vi "Vision Processing.vi"() -> ()   [LabVIEW 2011]
doc: "This VI runs in parallel to other tasks. It gets images from the camera, processes them for color or shape and use that information to affect robot behavior."
uses:
  Robot Global Data.vi
  <vilib>/vision/NI_Vision_Development_Module.lvlib
panel:
  out "Midpoint":dbl
  in  "Lower Speed Limit":dbl=0.05
  out "Turret Rotation":dbl
  in  "Upper Speed Limit":dbl=0.3
  out "Number of Rectangles Visible":dbl
  out "Y Position Array":dbl[](array[numeric])
  out "X Position Array":dbl[](array[numeric])
  out "Array":T1(array[cluster])
  in  "Score Limits":T2={"Rect Coverage"=76.0, "Aspect Ratio"=40.0, "X Edge Strength"=40.0, "Y Edge Strength"=60.0}
  out "Processed Image":T3(plugin-control)
  out "Original Image":T3(plugin-control)
  in  "Annotate":bool=TRUE
  in  "Particle Count Limit":i32=10
  in  "Area Size Limit":i32=444
  in  "Range":cluster{"Lower value":sgl, "Upper value":sgl}={"Lower value"=120.0, "Upper value"=255.0}
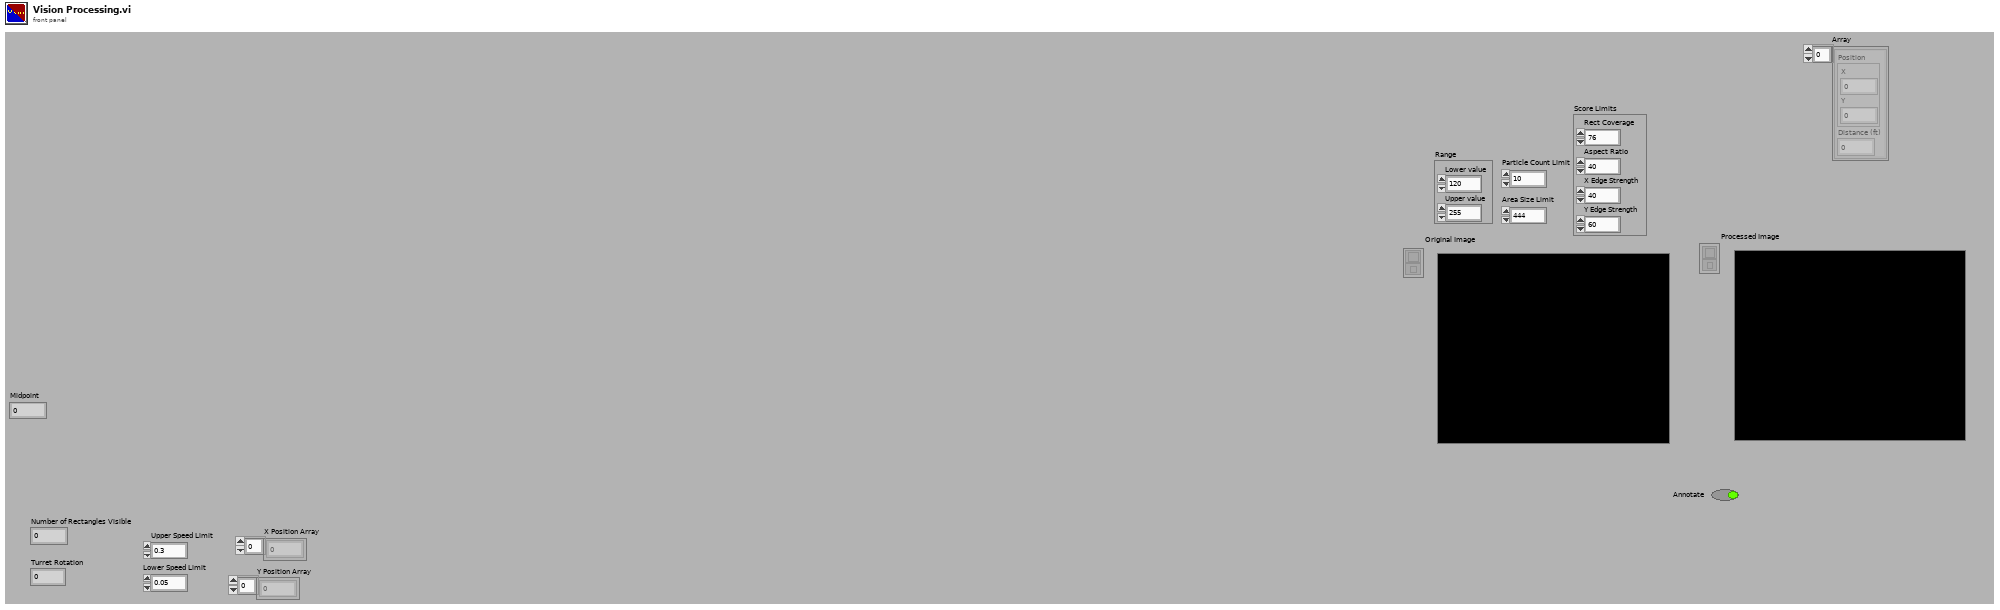
[diagram p1: front panel]
types:
  T1 = cluster{"Position":cluster{"X":dbl, "Y":dbl}, "Distance (ft)":dbl}[]
  T2 = cluster{"Rect Coverage":dbl, "Aspect Ratio":dbl, "X Edge Strength":dbl, "Y Edge Strength":dbl}
  T3 = typedef "IMAQ Image.ctl" = refnum<image>
  T4 = typedef "Image Type" = u32
  T5 = typedef "WPI_CameraImageSize.ctl" = enum16{"640x480", "320x240", "160x120"}
  T6 = cluster{"fps":i32, "compression":i32, "Image Size":T5}
  T7 = cluster{cluster{"Left":dbl, "Top":dbl, "Right":dbl, "Bottom":dbl}, dbl[]}[]
  T8 = cluster{"Left":dbl, "Top":dbl, "Right":dbl, "Bottom":dbl}
  T9 = cluster{"Target Center (-1 to 1)":cluster{"X":dbl, "Y":dbl}, "Distance (ft)":dbl}
  T10 = cluster{"Target Center (-1 to 1)":cluster{"X":dbl, "Y":dbl}, "Distance (ft)":dbl}[]
  T11 = cluster{"Axis 1":dbl, "Axis 2":dbl, "Axis 3":dbl, "Axis 4":dbl, "Axis 5":dbl, "Axis 6":dbl, "Button 1":bool, "Button 2":bool, "Button 3":bool, "Button 4":bool, "Button 5":bool, "Button 6":bool, "Button 7":bool, "Button 8":bool, "Button 9":bool, "Button 10":bool, "Button 11":bool, "Button 12":bool}
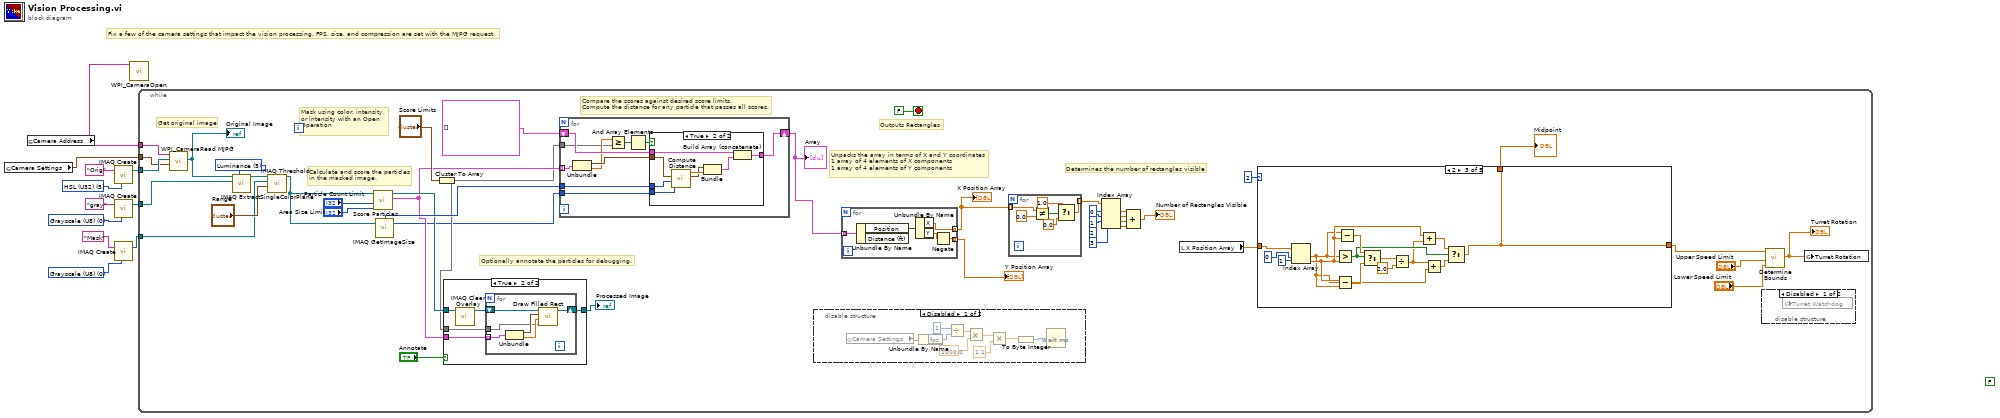
[diagram p0: block diagram]
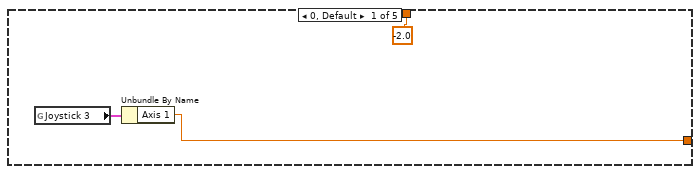
[diagram p4: hidden frame]
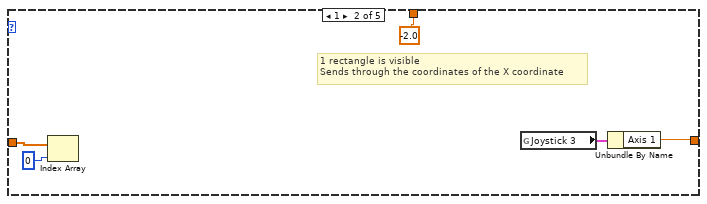
[diagram p5: hidden frame]
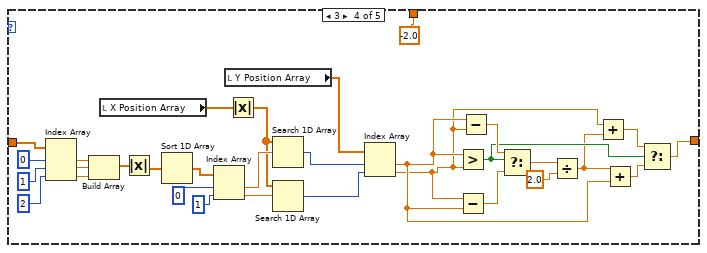
[diagram p6: hidden frame]
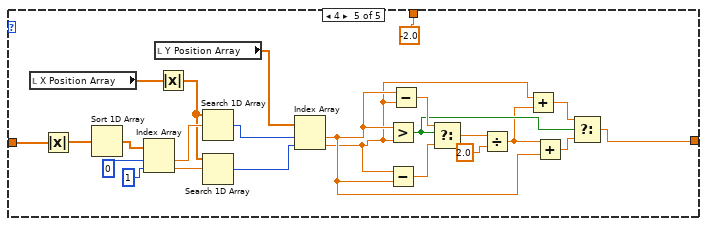
[diagram p7: hidden frame]
diagram:
  (unwired) FALSE
  w4 = T4 0 items=["Grayscale (U8)", "Grayscale (I16)", "Grayscale (SGL)", "Complex (CSG)", "RGB (U32)", "HSL (U32)", "RGB (U64)", "Grayscale (U16)"] ("Image Type")
  w8 = T4 5 items=["Grayscale (U8)", "Grayscale (I16)", "Grayscale (SGL)", "Complex (CSG)", "RGB (U32)", "HSL (U32)", "RGB (U64)", "Grayscale (U16)"] ("Image Type")
  w11 = T4 0 items=["Grayscale (U8)", "Grayscale (I16)", "Grayscale (SGL)", "Complex (CSG)", "RGB (U32)", "HSL (U32)", "RGB (U64)", "Grayscale (U16)"] ("Image Type")
  # "Fix a few of the camera settings that impact the vision processing. FPS, size, and compression are set with the MJPG request."
  n1 = global read "Robot Global Data.vi" "Camera Settings"() -> (w1:T6)
  n2 = global read "Robot Global Data.vi" "Camera Address"() -> (w2:string)
  n3 = call "IMAQ Create"("Image Name"="Orig", "Image Type"=w8) -> ("New Image"=w7:T3)  [unwired: 2 in, 2 out]
  n4 = call "IMAQ Create"("Image Name"="gray", "Image Type"=w11) -> ("New Image"=w6:T3)  [unwired: 2 in, 2 out]
  n5 = call "IMAQ Create"("Image Name"="Mask", "Image Type"=w4) -> ("New Image"=w3:T3)  [unwired: 2 in, 2 out]
  n6 = call <vilib>:"WPI_CameraOpen.vi"("Camera Address"=w2) -> ()  [unwired: 9 in, 2 out]
  n7 = while {
    tunnel: w7 -> [w52]
    tunnel: w6 -> [w34]
    tunnel: w3 -> [w36]
    tunnel: w2 -> [w51]
    tunnel: w1 -> [w40]
    stop <- FALSE stop-if-true
    w39 = 5 items=["Red", "Green", "Blue", "Hue", "Saturation", "Luminance", "Value", "Intensity"] ("Color Plane")
    # "Determines the number of rectangles visible"
    # "Unpacks the array in terms of X and Y coordinates\n1 array of 4 elements of X components\n1 array of 4 elements of Y components"
    # "Outputs Rectangles"
    # "Optionally annotate the particles for debugging."
    # "Compare the scores against desired score limits.\nCompute the distance for any particle that passes all scores."
    # "Calculate and score the particles\nin the masked image."
    # "Mask using color, intensity,\nor intensity with an Open\nOperation"
    # "Get original image"
    n8 = call <vilib>:"WPI_CameraRead MJPG.vi"("Camera Settings"=w40, "Image"=w52, "address"=w51) -> ("Image Out"=w35:T3)  [unwired: 7 in, 1 out]
    "Original Image" <- w35
    n9 = call "IMAQ ExtractSingleColorPlane"("Color Plane"=w39, "Image Dst"=w34, "Image Src"=w35) -> ("Image Dst Out"=w37:T3)  [unwired: 1 in, 7 out]
    n10 = call "IMAQ Threshold"("Range"="Range", "Image Dst"=w36, "Image Src"=w37) -> ("Image Dst Out"=w33:T3)  [unwired: 3 in, 5 out]
    n11 = call "Score Particles.vi"("Area Size Limit"="Area Size Limit", "Particle Count Limit"="Particle Count Limit", "Image Refnum in"=w33) -> ("Scored Particle Info"=w47:T7, "Image Refnum out"=w50:T3)  [unwired: 7 in]
    n12 = call "IMAQ GetImageSize"("Image"=w33) -> ("Y Resolution"=w41:i32, "X Resolution"=w53:i32)  [unwired: 3 in, 1 out]
    n13 = Cluster To Array(cluster="Score Limits") -> (array=w45:dbl[])
    n14 = case shown="True" "Annotate" {
      tunnel: w50 -> [w151 w156]
      tunnel: [w151 w155] -> w48
      tunnel: w47 -> [_ w153]
      tunnel: w45 -> [_ w152]
      frame False {
      }
      frame True {
        n15 = call "IMAQ Clear Overlay"("Image"=w156) -> ("Image Out"=w154:T3)  [unwired: 2 in, 8 out]
        n16 = for {
          shift-right: [w161] -> w155
          shift-left: w154 -> [w162]
          tunnel: w153 -> [w158] mode=indexing
          tunnel: w152 -> [w157]
          n17 = Unbundle(w158) -> (w159:T8, w160:dbl[])
          n18 = call "Draw Filled Rect.vi"("Limits"=w157, "Scores"=w160, "Bounding Box"=w159, "image in"=w162) -> ("image out"=w161:T3)  [unwired: 7 in]
        }
      }
    }
    "Processed Image" <- w48
    n19 = for {
      shift-right: [w171] -> w12
      shift-left: T1 [] -> [w172]
      tunnel: w53 -> [w170]
      tunnel: w47 -> [w168] mode=indexing
      tunnel: w45 -> [w164]
      tunnel: w41 -> [w163]
      n20 = Unbundle(w168) -> (w169:T8, w165:dbl[])
      n21 = Greater Or Equal?(x=w165, y=w164) -> (x >= y?=w167:bool[])
      n22 = And Array Elements(Boolean array=w167) -> (logical AND=w166:bool)
      n23 = case shown="True" w166 {
        tunnel: w172 -> [w173 w181]
        tunnel: [w173 w180] -> w171
        tunnel: w169 -> [_ w176]
        tunnel: w170 -> [_ w178]
        tunnel: w163 -> [_ w174]
        frame False {
        }
        frame True {
          n24 = call "Compute Distance.vi"("Y Image Resolution"=w174, "X Image Resolution"=w178, "Bounding Box"=w176) -> ("Target Center (-1 to 1)"=w175:cluster{"X":dbl, "Y":dbl}, "Distance (ft)"=w177:dbl)  [unwired: 7 in]
          n25 = Bundle("Target Center (-1 to 1)"=w175, "Distance (ft)"=w177) -> (w179:T9)  [unwired: 1 in]
          n26 = Build Array (concatenate)(w181, w179) -> (w180:T10)
        }
      }
    }
    "Array" <- w12
    n27 = disable-structure shown="Disabled" {
      frame Disabled {
        n28 = global read "Robot Global Data.vi" "Camera Settings"() -> (w54:T6)
        n29 = Unbundle By Name(w54) -> ("fps"=w55:i32)
        n30 = Divide(x=1, y=w55) -> (x/y=w57:dbl)
        n31 = Multiply(x=w57, y=1000.0) -> (x*y=w59:dbl)
        n32 = Multiply(x=w59, y=1.1) -> (x*y=w61:dbl)
        n33 = To Byte Integer(number=w61) -> (8bit integer=w62:i8)
        n34 = Wait (ms)(milliseconds to wait=w62) -> ()  [unwired: 1 out]
      }
      frame Enabled {
      }
    }
    n35 = for {
      tunnel: [w148] -> w25 mode=indexing
      tunnel: [w149] -> w14 mode=indexing
      tunnel: w12 -> [w146] mode=indexing
      n36 = Unbundle By Name(w146) -> ("Position"=w150:cluster{"X":dbl, "Y":dbl})  [unwired: 1 out]
      n37 = Unbundle By Name(w150) -> ("X"=w149:dbl, "Y"=w147:dbl)
      n38 = Negate(x=w147) -> (-x=w148:dbl)
    }
    "X Position Array" <- w14
    "Y Position Array" <- w25
    n39 = for {
      tunnel: w14 -> [w67] mode=indexing
      tunnel: [w63] -> w15 mode=indexing
      n40 = Not Equal?(x=w67, y=0.0) -> (x != y?=w66:bool)
      n41 = Select(t=1.0, s=w66, f=0.0) -> (s? t:f=w63:dbl)
    }
    n42 = Index Array(array=w15, index #1=0 ("index"), index #2=1 ("index"), index #3=2 ("index"), index #4=3 ("index")) -> (element #1=w17:dbl, element #2=w16:dbl, element #3=w18:dbl, element #4=w19:dbl)
    n43 = Compound Arithmetic op=ADD(w17, w16, w18, w19) -> (→"Number of Rectangles Visible":dbl)
    n44 = local read "X Position Array"() -> (w13:dbl[])
    n45 = case shown="2" 2 {
      tunnel: w13 -> [_ w76 w90 w121 w125]
      tunnel: [w70 w73 w77 w93 w124] -> w29
      tunnel: [-2.0 -2.0 w77 -2.0 -2.0] -> w30
      frame 0, Default {
        n46 = global read "Robot Global Data.vi" "Joystick 3"() -> (w71:T11)
        n47 = Unbundle By Name(w71) -> ("Axis 1"=w70:dbl)
      }
      frame 1 {
        # "1 rectangle is visible\nSends through the coordinates of the X coordinate"
        n48 = Index Array(array=w76, index=0) -> ()  [unwired: 1 out]
        n49 = global read "Robot Global Data.vi" "Joystick 3"() -> (w74:T11)
        n50 = Unbundle By Name(w74) -> ("Axis 1"=w73:dbl)
      }
      frame 2 {
        n51 = Index Array(array=w90, index #1=0 ("index"), index #2=1 ("index")) -> (element #1=w78:dbl, element #2=w79:dbl)
        n52 = Greater?(x=w78, y=w79) -> (0:w83:bool)
        n53 = Subtract(x=w79, y=w78) -> (x-y=w86:dbl)
        n54 = Subtract(x=w78, y=w79) -> (x-y=w87:dbl)
        n55 = Select(t=w87, s=w83, f=w86) -> (s? t:f=w85:dbl)
        n56 = Divide(x=w85, y=2.0) -> (x/y=w80:dbl)
        n57 = Add(x=w79, y=w80) -> (x+y=w82:dbl)
        n58 = Add(x=w80, y=w78) -> (x+y=w81:dbl)
        n59 = Select(t=w82, s=w83, f=w81) -> (s? t:f=w77:dbl)
      }
      frame 3 {
        n60 = Index Array(array=w121, index #1=0 ("index"), index #2=1 ("index"), index #3=2 ("index")) -> (element #1=w117:dbl, element #2=w116:dbl, element #3=w115:dbl)
        n61 = Build Array(w117, w116, w115) -> (w114:dbl[])
        n62 = local read "X Position Array"() -> (w107:dbl[])
        n63 = Absolute Value(x=w114) -> (abs(x)=w113:dbl[])
        n64 = Sort 1D Array(array=w113) -> (sorted array=w112:dbl[])
        n65 = Index Array(array=w112, index #1=0 ("index"), index #2=1 ("index")) -> (element #1=w109:dbl, element #2=w108:dbl)
        n66 = local read "Y Position Array"() -> (w105:dbl[])
        n67 = Absolute Value(x=w107) -> (abs(x)=w92:dbl[])
        n68 = Search 1D Array(1D array=w92, element=w109) -> (index of element=w106:i32)  [unwired: 1 in]
        n69 = Search 1D Array(1D array=w92, element=w108) -> (index of element=w104:i32)  [unwired: 1 in]
        n70 = Index Array(array=w105, index #1=w106, index #2=w104) -> (element #1=w95:dbl, element #2=w94:dbl)
        n71 = Greater?(x=w95, y=w94) -> (0:w99:bool)
        n72 = Subtract(x=w94, y=w95) -> (x-y=w102:dbl)
        n73 = Subtract(x=w95, y=w94) -> (x-y=w103:dbl)
        n74 = Select(t=w103, s=w99, f=w102) -> (s? t:f=w101:dbl)
        n75 = Divide(x=w101, y=2.0) -> (x/y=w96:dbl)
        n76 = Add(x=w94, y=w96) -> (x+y=w98:dbl)
        n77 = Add(x=w96, y=w95) -> (x+y=w97:dbl)
        n78 = Select(t=w98, s=w99, f=w97) -> (s? t:f=w93:dbl)
      }
      frame 4 {
        n79 = local read "X Position Array"() -> (w139:dbl[])
        n80 = Absolute Value(x=w125) -> (abs(x)=w145:dbl[])
        n81 = Sort 1D Array(array=w145) -> (sorted array=w144:dbl[])
        n82 = Index Array(array=w144, index #1=0 ("index"), index #2=1 ("index")) -> (element #1=w141:dbl, element #2=w140:dbl)
        n83 = local read "Y Position Array"() -> (w137:dbl[])
        n84 = Absolute Value(x=w139) -> (abs(x)=w123:dbl[])
        n85 = Search 1D Array(1D array=w123, element=w141) -> (index of element=w138:i32)  [unwired: 1 in]
        n86 = Search 1D Array(1D array=w123, element=w140) -> (index of element=w136:i32)  [unwired: 1 in]
        n87 = Index Array(array=w137, index #1=w138, index #2=w136) -> (element #1=w127:dbl, element #2=w126:dbl)
        n88 = Greater?(x=w127, y=w126) -> (0:w131:bool)
        n89 = Subtract(x=w126, y=w127) -> (x-y=w134:dbl)
        n90 = Subtract(x=w127, y=w126) -> (x-y=w135:dbl)
        n91 = Select(t=w135, s=w131, f=w134) -> (s? t:f=w133:dbl)
        n92 = Divide(x=w133, y=2.0) -> (x/y=w128:dbl)
        n93 = Add(x=w126, y=w128) -> (x+y=w130:dbl)
        n94 = Add(x=w128, y=w127) -> (x+y=w129:dbl)
        n95 = Select(t=w130, s=w131, f=w129) -> (s? t:f=w124:dbl)
      }
    }
    "Midpoint" <- w30
    n96 = disable-structure shown="Disabled" {
      frame Disabled {
        n97 = global read "Robot Global Data.vi" "Turret Watchdog"() -> ()  [unwired: 1 in]
      }
      frame Enabled {
      }
    }
    n98 = call "Determine Bounds.vi"("Lower Limit"="Lower Speed Limit", "Upper Limit"="Upper Speed Limit", "Input"=w29) -> ("Output"=w28:dbl)  [unwired: 8 in]
    "Turret Rotation" <- w28
    n99 = global write "Robot Global Data.vi" "Turret Rotation"(w28) -> ()
  }
